vi "Read Operation Complete Msg.vi"(11 "Generic Optimization in":refnum<class "Generic Optimization.lvclass">) -> (2 "Operation Complete Msg":refnum<class "Operation Complete Msg.lvclass">, 3 "Generic Optimization out":refnum<class "Generic Optimization.lvclass">)   [LabVIEW 2016]
uses:
  Generic Optimization.lvclass
  C:/Users/Administrator/Desktop/LabVIEW EMS/SCADA Sub Abstract Actor/SCADA Sub Abstract/SCADA Sub Abstract.lvclass
  C:/Users/Administrator/Desktop/LabVIEW EMS/EMS Generic Actor/EMS Generic/EMS Generic.lvclass
  C:/Program Files (x86)/National Instruments/LabVIEW 2016/vi.lib/ActorFramework/Actor/Actor.lvclass
  Generic Optimization Messages/Operation Complete Msg/Operation Complete Msg.lvclass
  C:/Program Files (x86)/National Instruments/LabVIEW 2016/vi.lib/ActorFramework/Message/Message.lvclass
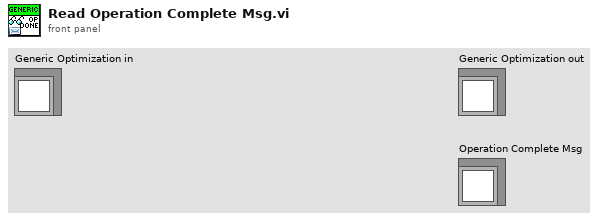
[diagram p1: front panel]
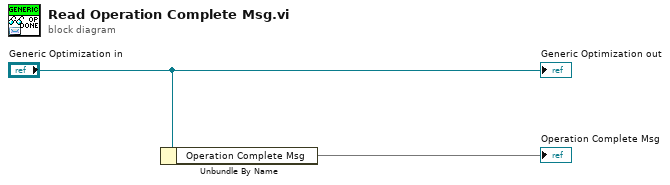
[diagram p0: block diagram]
diagram:
  n1 = Unbundle By Name("Generic Optimization in") -> ("Operation Complete Msg"=→"Operation Complete Msg")
  "Generic Optimization out" <- "Generic Optimization in"
